vi "CalculateCoordinates_171213.vi"(0 "X1":sgl, 1 "Y1":sgl, 2 "X2":sgl, 3 "Y2":sgl) -> (9 "x1-x2":sgl, 11 "y1-y2":sgl, 14 "sina":sgl, 15 "R from center":sgl, 16 "Mouse Xc":sgl, 17 "Mouse Yc":sgl, 18 "Cage Xc":sgl, 19 "Cage Yc":sgl)   [LabVIEW 2016]
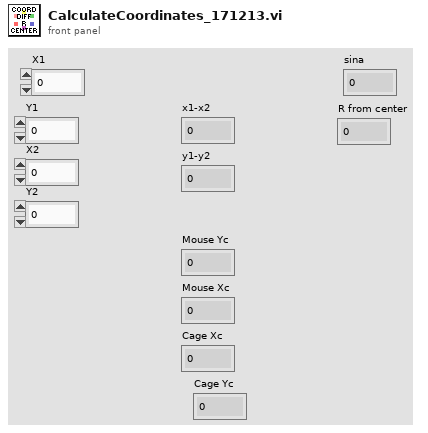
[diagram p1: front panel]
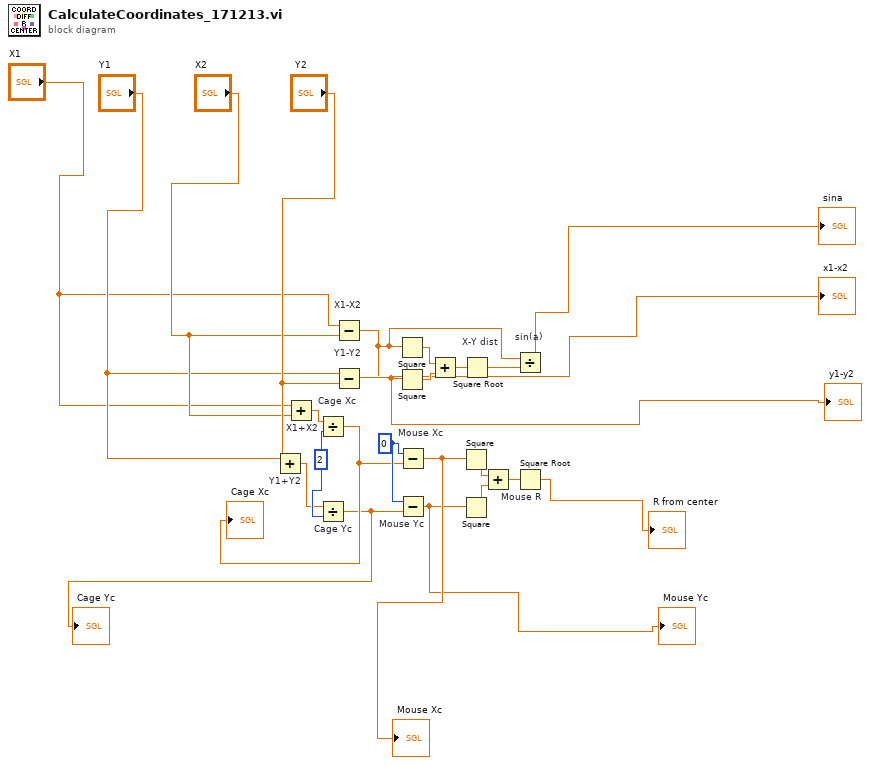
[diagram p0: block diagram]
diagram:
  w13 = 0
  w16 = 2
  n1 = Add "Y1+Y2"(x="Y1", y="Y2") -> (x+y=w15:sgl)
  n2 = Add "X1+X2"(x="X1", y="X2") -> (x+y=w14:sgl)
  n3 = Divide "Cage Xc"(x=w14, y=w16) -> (x/y=w12:sgl)
  "Cage Xc" <- w12
  n4 = Divide "Cage Yc"(x=w15, y=w16) -> (x/y=w11:sgl)
  "Cage Yc" <- w11
  n5 = Subtract "X1-X2"(x="X1", y="X2") -> (x-y=w6:sgl)
  "x1-x2" <- w6
  n6 = Subtract "Y1-Y2"(x="Y1", y="Y2") -> (x-y=w7:sgl)
  "y1-y2" <- w7
  n7 = Square(x=w6) -> (x^2=w17:sgl)
  n8 = Square(x=w7) -> (x^2=w18:sgl)
  n9 = Subtract "Mouse Xc"(x=w13, y=w12) -> (x-y=w10:sgl)
  "Mouse Xc" <- w10
  n10 = Subtract "Mouse Yc"(x=w13, y=w11) -> (x-y=w9:sgl)
  "Mouse Yc" <- w9
  n11 = Add(x=w17, y=w18) -> (x+y=w19:sgl)
  n12 = Square(x=w10) -> (x^2=w21:sgl)
  n13 = Square(x=w9) -> (x^2=w22:sgl)
  n14 = Square Root "X-Y dist"(x=w19) -> (sqrt(x)=w20:sgl)
  n15 = Add(x=w21, y=w22) -> (x+y=w23:sgl)
  n16 = Divide "sin(a)"(x=w6, y=w20) -> (x/y=→"sina":sgl)
  n17 = Square Root "Mouse R"(x=w23) -> (sqrt(x)=→"R from center":sgl)
